vi "PH_VacuumControl.Set Status.vi"(0 "i ref in":refnum<vi>, 2 "Status":T1 caption="Enabling State" items=["no info", "off/false/out", "on/true/in", "Failure", "Alarm", "Status 1", "Status 2", "Status 3"], 5 "error in (no error)":errorcluster) -> (14 "i ref out":refnum<vi>, 19 "error out":errorcluster)   [LabVIEW 2014, in "PH_VacuumControl.lvlib"]
doc: "This VI sets the device state to own attributes, to the related GUI element and to the related memory tag, if the incoming state differs from the one stored in own attributes."
uses:
  PH_VacuumControl.lvlib
  PH_StatusHandler/PH_StatusHandler.Status.ctl
  PH_Common/PH_Common.lvlib
  PH_StatusHandler/PH_StatusHandler.lvlib
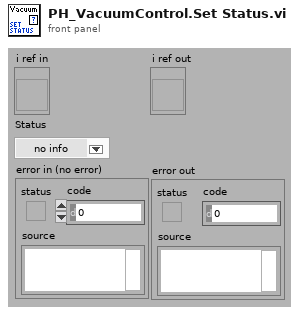
[diagram p1: front panel]
types:
  T1 = typedef "PH_StatusHandler.lvlib/PH_StatusHandler.Status.ctl" = i16
  T2 = typedef "PH_VacuumControl.lvlib/PH_VacuumControl.i attribute.ctl" = cluster{"GUI Refs":cluster{"Exit":refnum<vi>, "Set Unit":refnum<vi>, "Device found":refnum<vi>, "Busy":refnum<vi>, "State":refnum<vi>, "Delete":refnum<vi>, "Channels":refnum<vi>, "Channel Name":refnum<vi>, "Trend":refnum<vi>, "Logarithmic":refnum<vi>, "Limit reached":refnum<vi>, "Channel Name 1 MT":refnum<vi>, "Channel Name 2 MT":refnum<vi>, "Trend MT":refnum<vi>, "Logarithmic MT":refnum<vi>, "Limit reached MT":refnum<vi>}, "Device found":bool, "Busy":bool, "Selected Unit":i32, "Channels [mbar]":T3, "Channel Names":cluster{"Channel 1":string, "Channel 2":string, "Channel 3":string, "Channel 4":string, "Channel 5":string, "Channel 6":string}, "Status":T1, "AGCxxx VISA Cluster":T4, "Instr Firmware Revision":string, "Service IDs Pressure":cluster{"Channel 1":i32, "Channel 2":i32, "Channel 3":i32, "Channel 4":i32, "Channel 5":i32, "Channel 6":i32}, "Service IDs Limits":cluster{"Channel 1":i32, "Channel 2":i32, "Channel 3":i32, "Channel 4":i32, "Channel 5":i32, "Channel 6":i32}, "Trend":cluster{"Start Point":timestamp, "Pressures [mbar] Channel 1":dbl[], "Pressures [mbar] Channel 2":dbl[], "Pressures [mbar] Channel 3":dbl[], "Pressures [mbar] Channel 4":dbl[], "Pressures [mbar] Channel 5":dbl[], "Pressures [mbar] Channel 6":dbl[], "Timebase [s]":i32[], "Trend Channel":u16, "Start Fit":dbl, "Trend Channel 1 MT":u16, "Trend Channel 2 MT":u16, "Start or continue Fit MT":dbl, "Continue or start Fit MT":dbl, "Datasets strored":i32, "Dataarray Size":i32}, "Running":bool}
  T3 = typedef "PH_VacuumControl.lvlib/PH_VacuumControl.Channels.ctl" = cluster{"Channel 1":dbl, "Channel 2":dbl, "Channel 3":dbl, "Channel 4":dbl, "Channel 5":dbl, "Channel 6":dbl, "Name Channel 1":string, "Name Channel 2":string, "Name Channel 3":string, "Name Channel 4":string, "Name Channel 5":string, "Name Channel 6":string, "Upper Limit":dbl, "Upper Limit 2":dbl, "Upper Limit 3":dbl, "Upper Limit 4":dbl, "Upper Limit 5":dbl, "Upper Limit 6":dbl}
  T4 = typedef "AGCxxx - Driver.lvlib/AGCxxx VISA Control.ctl" = cluster{"VISA resource name":refnum<visa-resource-name>, "VISA Timeout Value (1000 ms)":u32, "Lock Timeout (1000 ms)":u32, "MAX Channel (6)":i32}
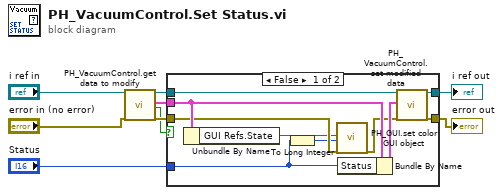
[diagram p0: block diagram]
diagram:
  n1 = call "PH_VacuumControl.get data to modify.vi"("i ref in"="i ref in", "error in (no error)"="error in (no error)") -> ("i ref out"=w4:refnum<vi>, "i attribute"=w2:T2, "timed out"=w3:bool, "error out"=w9:errorcluster)  [unwired: 14 in]
  n2 = case shown="False" w3 {
    tunnel: w9 -> [w15 w20]
    tunnel: [w19 w20] -> w8
    tunnel: [w18 w21] -> w6
    tunnel: w4 -> [w13 w21]
    tunnel: w2 -> [w17 _]
    tunnel: "Status" -> [w12 _]
    frame False {
      n3 = Unbundle By Name(w17) -> ("GUI Refs.State"=w11:refnum<vi>)
      n4 = To Long Integer(number=w12) -> (32bit integer=w10:i32)
      n5 = call "PH_GUI.set color GUI object.vi"("GUI object Ref"=w11, "State"=w10, "error in (no error)"=w15) -> ("error out"=w14:errorcluster)  [unwired: 16 in]
      n6 = Bundle By Name(cluster=w17, "Status"=w12) -> (w16:T2)
      n7 = call "PH_VacuumControl.set modified data.vi"("i ref in"=w13, "i attribute"=w16, "error in (no error)"=w14) -> ("i ref out"=w18:refnum<vi>, "error out"=w19:errorcluster)  [unwired: 15 in]
    }
    frame True {
    }
  }
  "error out" <- w8
  "i ref out" <- w6
